vi "TSM Clear DAQmx Tasks.vi"(0 "TSM context":T1) -> (15 "error out":errorcluster)   [LabVIEW 2019]
doc: "Use this VI to reset and clear all tasks for all NI-DAQmx instruments in the Semiconductor Module Context."
uses:
  <vilib>/NI_TestStand_SemiconductorModule/NI_TestStand_Semiconductor_Module.lvlibp/PinMap/General/SemiconductorModuleContext.ctl
  <vilib>/NI_TestStand_SemiconductorModule/NI_TestStand_Semiconductor_Module.lvlibp
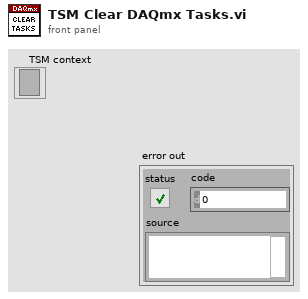
[diagram p1: front panel]
types:
  T1 = typedef "NI_TestStand_Semiconductor_Module.lvlibp/SemiconductorModuleContext.ctl" = refnum<k7>
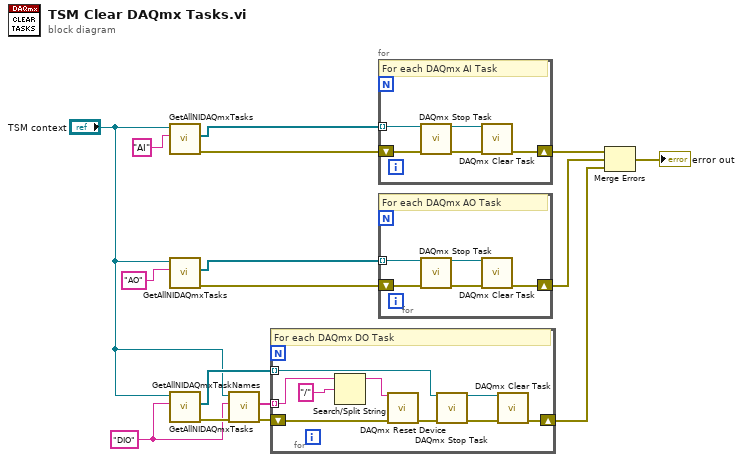
[diagram p0: block diagram]
diagram:
  w1 = "DIO" ("Task Type")
  n1 = call <vilib>:"GetAllNIDAQmxTasks.vi"("Task Type"="AI", "Semiconductor Module Context"="TSM context") -> ("error out"=w14:errorcluster, "DAQmx Tasks"=w16:refnum<k21>[])  [unwired: 7 in, 1 out]
  n2 = call <vilib>:"GetAllNIDAQmxTasks.vi"("Task Type"="AO", "Semiconductor Module Context"="TSM context") -> ("error out"=w11:errorcluster, "DAQmx Tasks"=w10:refnum<k21>[])  [unwired: 7 in, 1 out]
  n3 = call <vilib>:"GetAllNIDAQmxTasks.vi"("Task Type"=w1, "Semiconductor Module Context"="TSM context") -> ("error out"=w5:errorcluster, "DAQmx Tasks"=w7:refnum<k21>[])  [unwired: 7 in, 1 out]
  n4 = call <vilib>:"GetAllNIDAQmxTaskNames.vi"("error in (no error)"=w5, "Task Type"=w1, "Semiconductor Module Context"="TSM context") -> ("error out"=w4:errorcluster, "Channel Lists"=w3:string[])  [unwired: 5 in, 2 out]
  n5 = for {
    tunnel: w7 -> [w20] mode=indexing
    shift-right: [w24] -> w6
    shift-left: w4 -> [w22]
    tunnel: w3 -> [w18] mode=indexing
    # "For each DAQmx DO Task"
    n6 = Search/Split String(string=w18, search string/char (-)="/") -> (substring before match=w17:string)  [unwired: 1 in, 2 out]
    n7 = call <vilib>:"DAQmx Reset Device.vi"("device in"=w17, "error in"=w22) -> ("error out"=w21:errorcluster)  [unwired: 13 in]
    n8 = call <vilib>:"DAQmx Stop Task.vi"("task/channels in"=w20, "error in"=w21) -> ("task out"=w25:refnum<k21>, "error out"=w23:errorcluster)  [unwired: 12 in]
    n9 = call <vilib>:"DAQmx Clear Task.vi"("task in"=w25, "error in"=w23) -> ("error out"=w24:errorcluster)  [unwired: 13 in]
  }
  n10 = for {
    tunnel: w16 -> [w29] mode=indexing
    shift-right: [w27] -> w15
    shift-left: w14 -> [w30]
    # "For each DAQmx AI Task"
    n11 = call <vilib>:"DAQmx Stop Task.vi"("task/channels in"=w29, "error in"=w30) -> ("task out"=w28:refnum<k21>, "error out"=w26:errorcluster)  [unwired: 12 in]
    n12 = call <vilib>:"DAQmx Clear Task.vi"("task in"=w28, "error in"=w26) -> ("error out"=w27:errorcluster)  [unwired: 13 in]
  }
  n13 = for {
    tunnel: w10 -> [w34] mode=indexing
    shift-right: [w32] -> w8
    shift-left: w11 -> [w35]
    # "For each DAQmx AO Task"
    n14 = call <vilib>:"DAQmx Stop Task.vi"("task/channels in"=w34, "error in"=w35) -> ("task out"=w33:refnum<k21>, "error out"=w31:errorcluster)  [unwired: 12 in]
    n15 = call <vilib>:"DAQmx Clear Task.vi"("task in"=w33, "error in"=w31) -> ("error out"=w32:errorcluster)  [unwired: 13 in]
  }
  n16 = Merge Errors(w15, w8, w6) -> (→"error out":errorcluster)
